vi "Multi-Selection-Dialog-Box.vi"(3 "Start In":path=path "D:/", 4 "Group":refnum<vi>, 5 "cluster in":T1={"Kinetics"=[], "Spectrum"=[], "Experiments groups"=[], "GRAPH EXPERIMENTAL DATA"=[], "error out"={"status"=FALSE, "code"=0, "source"=""}, "group"=0, "exp selected"=0, "# exp"=0, "kinetics plot names"=[], "spectra plot names"=[], "FromToWave"={"FromWave"=0.0, "ToWave"=0.0}, "Laser shutter task"="", "Accelerator task"="", "Motor task"="", "GRAPH EXPERIMENTAL DATA ref"=refnum, "timedelays"=[0.0, 0.0, 0.0, 0.0, 0.0, 0.0, 0.0, 0.06019061100911815, 0.0521779104562645, 0.045231877429679615, 0.03921051490799832, 0.033990728811568754, 0.029465811603150715, 0.025543260876973825, 0.02214288834180205, 0.01919518054014414, 0.016639877791965713, 0.014424742312398925, 0.012504490320209958, 0.010839866306230088, 0.009396840537117498, 0.008145913389103785, 0.00706151229029317, 0.006121468943269439, 0.005306566140927374, 0.004600144911132549, 0.003987763959109073, 0.0034569044455719407, 0.00299671406541447, 0.0025977851951783253, 0.0022519625739982996, 0.00195217658646366, 0.0016922987392150965, 0.0014670163768006634, 0.0012717240756200802, 0.0011024294957352762, 0.0009556717658856477, 0.0008284507332614981, 0.0007181656316962257, 0.0006225619144775864, 0.0005396851648867825, 0.00046784114226338394, 0.0004055611468220084, 0.0003515719951773376, 0.00030476999279031153, 0.00026419837125694315, 0.00022902772919263772, 0.0001985390768670671, 0.0001721091379728629, 0.00014919760805372974, 0.00012933610911736794], "wavelengths"=[0.0, 0.0, 0.0, 0.0, 0.0, 0.0, 0.0, 0.06019061100911815, 0.0521779104562645, 0.045231877429679615, 0.03921051490799832, 0.033990728811568754, 0.029465811603150715, 0.025543260876973825, 0.02214288834180205, 0.01919518054014414, 0.016639877791965713, 0.014424742312398925, 0.012504490320209958, 0.010839866306230088, 0.009396840537117498, 0.008145913389103785, 0.00706151229029317, 0.006121468943269439, 0.005306566140927374, 0.004600144911132549, 0.003987763959109073, 0.0034569044455719407, 0.00299671406541447, 0.0025977851951783253, 0.0022519625739982996, 0.00195217658646366, 0.0016922987392150965, 0.0014670163768006634, 0.0012717240756200802, 0.0011024294957352762, 0.0009556717658856477, 0.0008284507332614981, 0.0007181656316962257, 0.0006225619144775864, 0.0005396851648867825, 0.00046784114226338394, 0.0004055611468220084, 0.0003515719951773376, 0.00030476999279031153, 0.00026419837125694315, 0.00022902772919263772, 0.0001985390768670671, 0.0001721091379728629, 0.00014919760805372974, 0.00012933610911736794], "Experiment"=refnum, "Commentaires exp"=refnum, "FromToDelay"={"FromDelay"=0.0, "ToDelay"=0.0}}) -> (0 "cancelled?":bool, 1 "String File Names":string[](array[string]), 2 "cluster out":T1={"Kinetics"=[], "Spectrum"=[], "Experiments groups"=[], "GRAPH EXPERIMENTAL DATA"=[], "error out"={"status"=FALSE, "code"=0, "source"=""}, "group"=0, "exp selected"=0, "# exp"=0, "kinetics plot names"=[], "spectra plot names"=[], "FromToWave"={"FromWave"=0.0, "ToWave"=0.0}, "Laser shutter task"="", "Accelerator task"="", "Motor task"="", "GRAPH EXPERIMENTAL DATA ref"=refnum, "timedelays"=[0.0, 0.0, 0.0, 0.0, 0.0, 0.0, 0.0, 0.06019061100911815, 0.0521779104562645, 0.045231877429679615, 0.03921051490799832, 0.033990728811568754, 0.029465811603150715, 0.025543260876973825, 0.02214288834180205, 0.01919518054014414, 0.016639877791965713, 0.014424742312398925, 0.012504490320209958, 0.010839866306230088, 0.009396840537117498, 0.008145913389103785, 0.00706151229029317, 0.006121468943269439, 0.005306566140927374, 0.004600144911132549, 0.003987763959109073, 0.0034569044455719407, 0.00299671406541447, 0.0025977851951783253, 0.0022519625739982996, 0.00195217658646366, 0.0016922987392150965, 0.0014670163768006634, 0.0012717240756200802, 0.0011024294957352762, 0.0009556717658856477, 0.0008284507332614981, 0.0007181656316962257, 0.0006225619144775864, 0.0005396851648867825, 0.00046784114226338394, 0.0004055611468220084, 0.0003515719951773376, 0.00030476999279031153, 0.00026419837125694315, 0.00022902772919263772, 0.0001985390768670671, 0.0001721091379728629, 0.00014919760805372974, 0.00012933610911736794], "wavelengths"=[0.0, 0.0, 0.0, 0.0, 0.0, 0.0, 0.0, 0.06019061100911815, 0.0521779104562645, 0.045231877429679615, 0.03921051490799832, 0.033990728811568754, 0.029465811603150715, 0.025543260876973825, 0.02214288834180205, 0.01919518054014414, 0.016639877791965713, 0.014424742312398925, 0.012504490320209958, 0.010839866306230088, 0.009396840537117498, 0.008145913389103785, 0.00706151229029317, 0.006121468943269439, 0.005306566140927374, 0.004600144911132549, 0.003987763959109073, 0.0034569044455719407, 0.00299671406541447, 0.0025977851951783253, 0.0022519625739982996, 0.00195217658646366, 0.0016922987392150965, 0.0014670163768006634, 0.0012717240756200802, 0.0011024294957352762, 0.0009556717658856477, 0.0008284507332614981, 0.0007181656316962257, 0.0006225619144775864, 0.0005396851648867825, 0.00046784114226338394, 0.0004055611468220084, 0.0003515719951773376, 0.00030476999279031153, 0.00026419837125694315, 0.00022902772919263772, 0.0001985390768670671, 0.0001721091379728629, 0.00014919760805372974, 0.00012933610911736794], "Experiment"=refnum, "Commentaires exp"=refnum, "FromToDelay"={"FromDelay"=0.0, "ToDelay"=0.0}})   [LabVIEW 2015]
doc: "This VI allows you to use the Multiple Selection Dialog Box example and shows how to use it. Below is a description of each of the controls that you will find in this VI:\n\n- Start in: The path that is passed into this VI that it looks in at the beginning of the run.\n- Files of Type: A 2D array of strings that lists the types of the files that you want to select from. Use it as follows: in the first column, enter the different limiting strings that you want to be able to pick from and in the second column, enter the name that you want to appear in the Files of Type control in the dialog box. For example, to be able to select either VIs and VI libraries or text files, your 2D array would look like the following:\n\n *.vi;*.llb VIs and Libraries\n *.txt Text Files\n\nNotice that if you want to enter multiple file types in the same string, you should separate them by a semicolon and make sure you do not include any spaces.\n- Window Title: The title of the dialog box that you want the user to see.\n- Path File Names: An array of paths that lists all the files that you selected.\n- String File Names: An array of strings that lists all the files that you selected.\n- Cancelled?: A boolean that determines whether the user pressed the Cancel button."
uses:
  controls/control-cluster.ctl
  Classes/Experiments_group.lvclass
panel:
  in  "Window Title":string="Select Files:"
  in  "Files of Type":string[][](array[string])=[["*.dat", "DAT"], ["*.img", "Streak"], ["*.txt", "txt"], ["*.*", "All Files"]]
  # "This VI shows you how to use the Multiple File Selection\nDialog Box example. Look in Show VI Info... from the Windows\nmenu to find out how to use it or show the help window\n(Ctrl-H) and point to the individual Controls to see what they are."
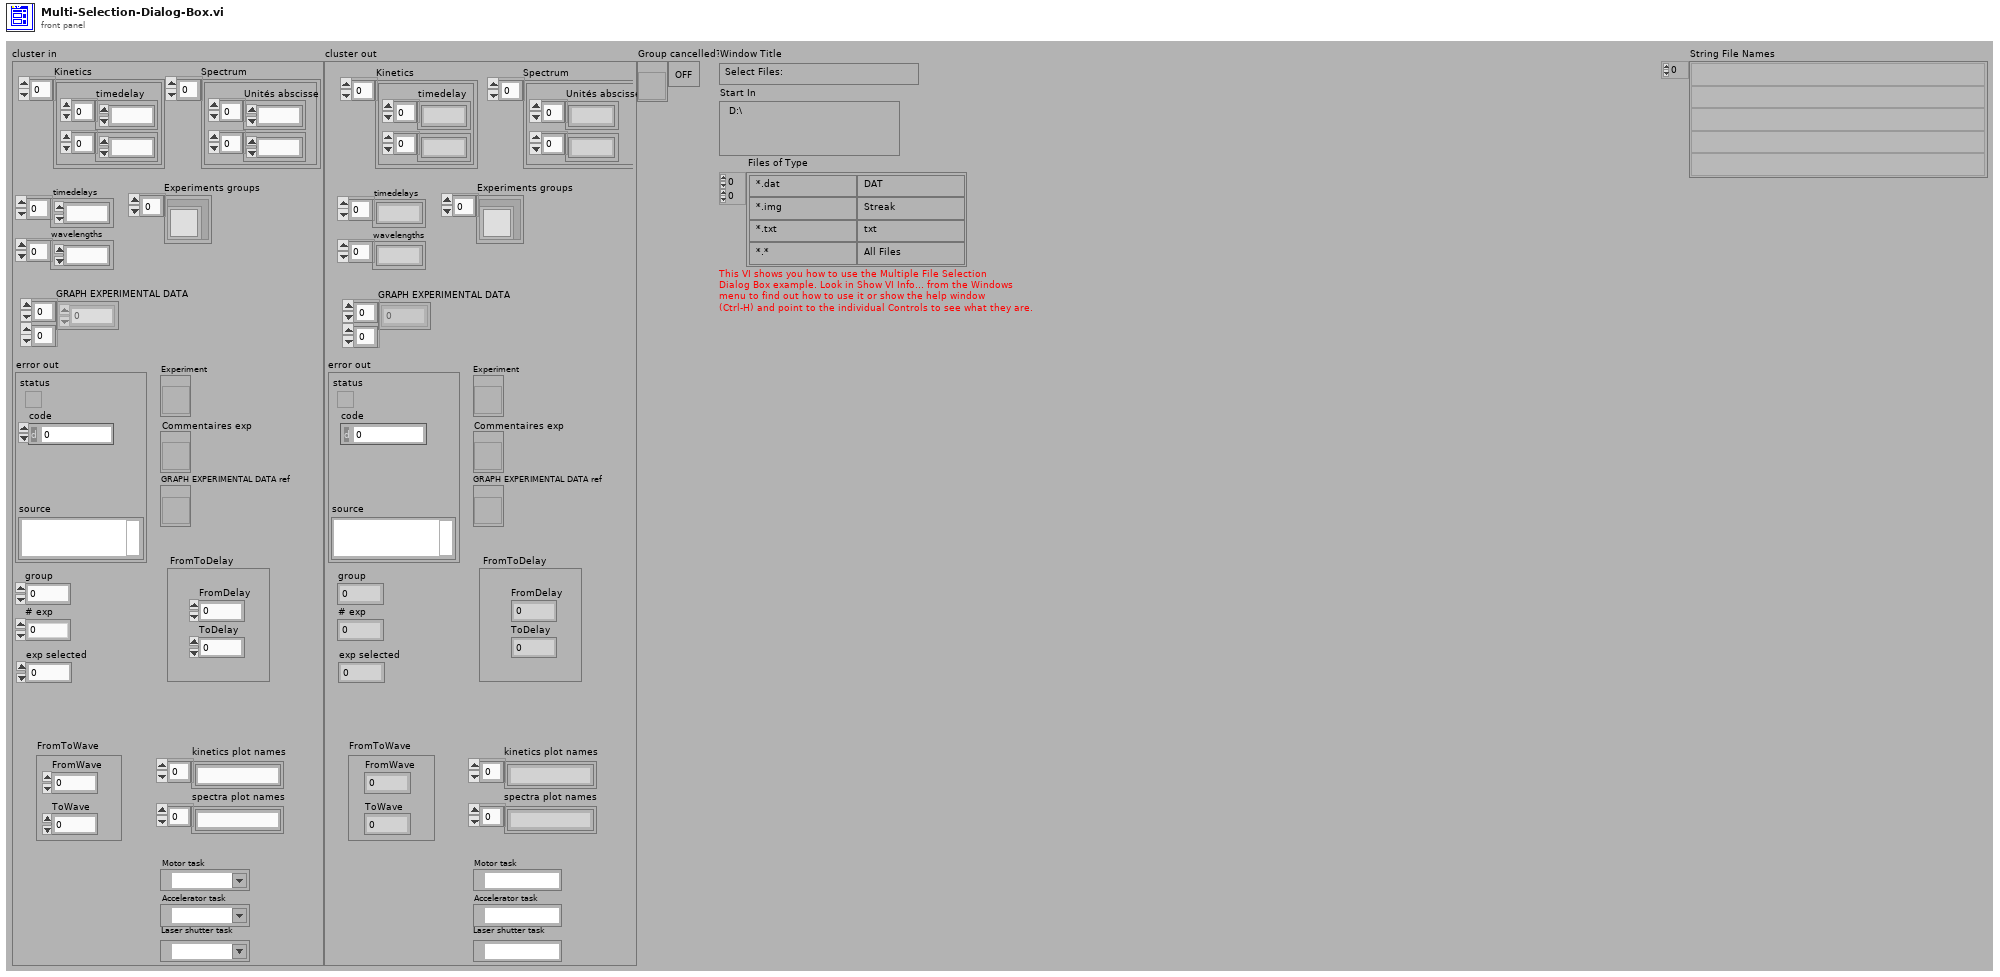
[diagram p1: front panel]
types:
  T1 = typedef "control-cluster.ctl" = cluster{"Kinetics":cluster{"timedelay":dbl[], dbl[]}[], "Spectrum":cluster{"Unités abscisse":dbl[], dbl[]}[], "Experiments groups":refnum<class "Experiments_group.lvclass">[], "GRAPH EXPERIMENTAL DATA":dbl[][], "error out":errorcluster, "group":i32, "exp selected":i32, "# exp":i32, "kinetics plot names":string[], "spectra plot names":string[], "FromToWave":cluster{"FromWave":dbl, "ToWave":dbl}, "Laser shutter task":refnum<k21>, "Accelerator task":refnum<k21>, "Motor task":refnum<k21>, "GRAPH EXPERIMENTAL DATA ref":refnum<vi>, "timedelays":dbl[], "wavelengths":dbl[], "Experiment":refnum<vi>, "Commentaires exp":refnum<vi>, "FromToDelay":cluster{"FromDelay":dbl, "ToDelay":dbl}}
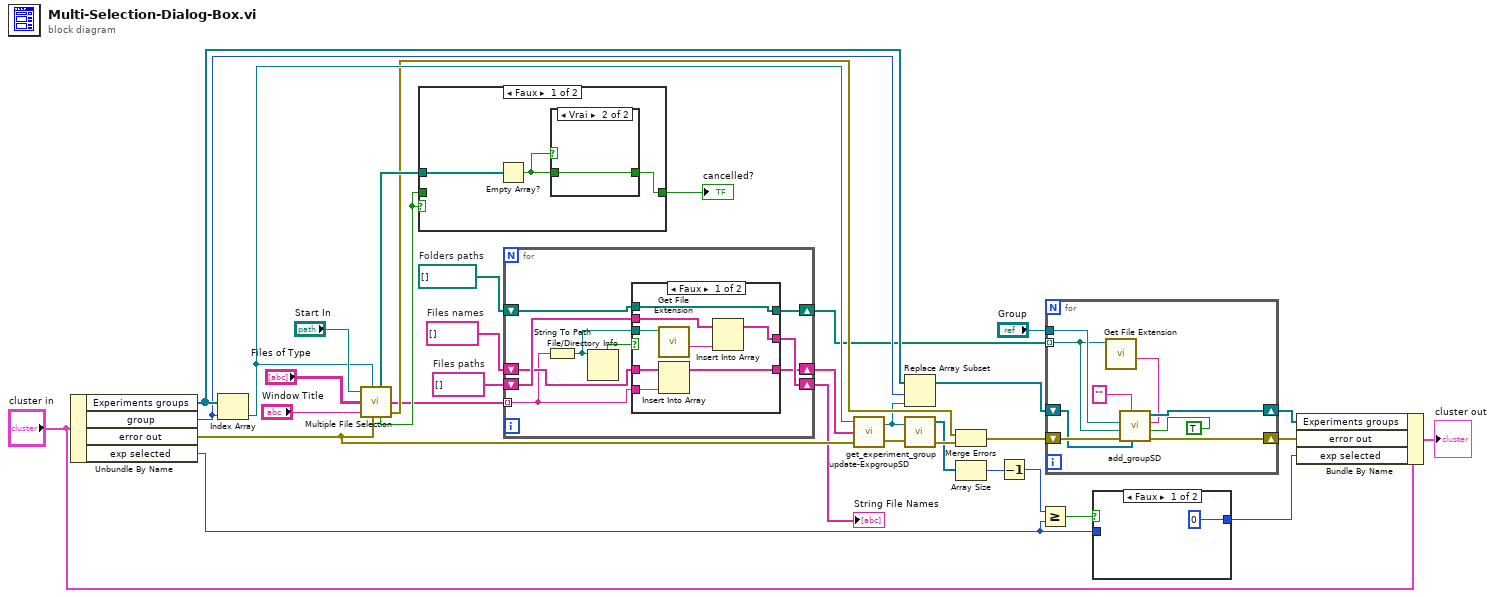
[diagram p0: block diagram]
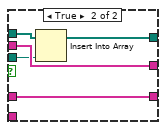
[diagram p3: hidden frame]
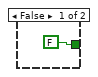
[diagram p4: hidden frame]
diagram:
  w17 = path[] []  # Folders paths
  w19 = string[] []  # Files names
  w21 = string[] []  # Files paths
  n1 = Unbundle By Name("cluster in") -> ("Experiments groups"=w28:refnum<class "Experiments_group.lvclass">[], "group"=w27:i32, "error out"=w24:errorcluster, "exp selected"=w2:i32)
  n2 = Index Array(array=w28, index=w27) -> (element=w25:refnum<class "Experiments_group.lvclass">)
  n3 = call "Multiple File Selection.vi"("Start In"="Start In", "EXP group IN"=w25, "Files of Type In"="Files of Type", "Window Title"="Window Title", "error in"=w24) -> ("Path File Names OUT"=w29:path[], "String File Names"=w22:string[], "cancelled?"=w31:bool, "error out"=w23:errorcluster)  [unwired: 1 in]
  n4 = case shown="Faux" w31 {
    tunnel: [w36 w40] -> w30
    tunnel: w31 -> [_ w40]
    tunnel: w29 -> [w37 _]
    frame False {
      n5 = Empty Array?(array=w37) -> (empty?=w35:bool)
      n6 = case shown="Vrai" w35 {
        tunnel: [FALSE w39] -> w36
        tunnel: w35 -> [_ w39]
        frame False {
        }
        frame True {
        }
      }
    }
    frame True {
    }
  }
  "cancelled?" <- w30
  n7 = for {
    tunnel: w22 -> [w43] mode=indexing
    shift-right: [w47] -> w20
    shift-left: w21 -> [w46]
    shift-right: [w45] -> w18
    shift-left: w19 -> [w44]
    shift-right: [w41] -> w10
    shift-left: w17 -> [w42]
    n8 = String To Path(string=w43) -> (path=w49:path)
    n9 = File/Directory Info(path=w49) -> (directory=w48:bool)  [unwired: 1 in, 6 out]
    n10 = case shown="Faux" w48 {
      tunnel: w49 -> [w57 w58]
      tunnel: [w55 w62] -> w47
      tunnel: w46 -> [w56 w62]
      tunnel: [w51 w61] -> w45
      tunnel: w44 -> [w53 w61]
      tunnel: w43 -> [w52 _]
      tunnel: w42 -> [w50 w60]
      tunnel: [w50 w59] -> w41
      frame False {
        n11 = call <vilib>:"Get File Extension.vi"("file"=w57) -> ("filename without extension"=w54:string)  [unwired: 6 in, 4 out]
        n12 = Insert Into Array(array=w53, new element=w52) -> (w51:string[])  [unwired: 1 in]
        n13 = Insert Into Array(array=w56, new element=w54) -> (w55:string[])  [unwired: 1 in]
      }
      frame True {
        n14 = Insert Into Array(array=w60, new element=w58) -> (w59:path[])  [unwired: 1 in]
      }
    }
  }
  "String File Names" <- w20
  n15 = call "update-ExpgroupSD.vi"("error in"=w24, "String File Paths"=w18, "EXP group"=w25) -> ("error out"=w8:errorcluster, "EXP group out"=w9:refnum<class "Experiments_group.lvclass">)
  n16 = Replace Array Subset(array=w28, new element=w9, index=w27) -> (w12:refnum<class "Experiments_group.lvclass">[])
  n17 = call-dynamic "get_experiment_group.vi"("Experiments_group.lvclass in"=w9, "error in (no error)"=w8) -> ("Experiments"=w6:refnum<class "Experiment.lvclass">[], "error out"=w7:errorcluster)  [unwired: 1 out]
  n18 = Merge Errors(w23, w7) -> (w14:errorcluster)
  n19 = Array Size(array=w6) -> (size(s)=w5:i32)
  n20 = Decrement(x=w5) -> (x-1=w4:i32)
  n21 = Greater Or Equal?(x=w4, y=w2) -> (x >= y?=w3:bool)
  n22 = for {
    tunnel: "Group" -> [w71]
    shift-right: [w68] -> w13
    shift-left: w14 -> [w69]
    shift-right: [w66] -> w11
    shift-left: w12 -> [w67]
    tunnel: w10 -> [w64] mode=indexing
    n23 = call <vilib>:"Get File Extension.vi"("file"=w64) -> ("filename without extension"=w63:string)  [unwired: 6 in, 4 out]
    n24 = call "add_groupSD.vi"("Upload"=TRUE, "Name group"=w63, "Experiments groups in"=w67, "Commentaires group"="", "error in (no error)"=w69, "Folder path"=w64, "group"=w71) -> ("error out"=w68:errorcluster, "Experiments groups out"=w66:refnum<class "Experiments_group.lvclass">[])  [unwired: 1 in]
  }
  n25 = case shown="Faux" w3 {
    tunnel: w2 -> [_ w73]
    tunnel: [0 w73] -> w1
    frame False {
    }
    frame True {
    }
  }
  n26 = Bundle By Name(cluster="cluster in", "Experiments groups"=w11, "error out"=w13, "exp selected"=w1) -> (→"cluster out":T1)
